vi "Data to XY Plot GPIB.vi"(7 "String of Data":string) -> (8 "XY Graph":cluster{sgl[], sgl[]}(graph))   [LabVIEW 2024, in "Keithley 648X Series.lvlib"]
doc: "Sends a default command string to the instrument whenever a new VISA session is opened, or the instrument is reset. Use this VI as a subVI for the <b>Initialize</b> and <b>Reset</b> VIs. Altering this VI could cause these two VIs to operate incorrectly."
uses:
  <instrlib>/Keithley 648X Series/Keithley 648X Series.lvlib
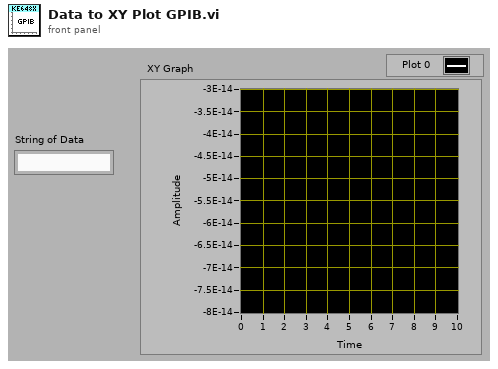
[diagram p1: front panel]
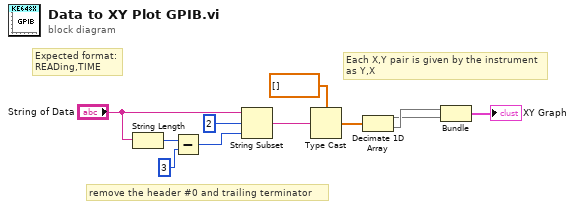
[diagram p0: block diagram]
diagram:
  # "remove the header #0 and trailing terminator"
  # "Each X,Y pair is given by the instrument\nas Y,X"
  # "Expected format:\nREADing,TIME"
  n1 = String Length(string="String of Data") -> (length=w11:i32)
  n2 = Subtract(x=w11, y=3) -> (x-y=w7:i32)
  n3 = String Subset(string="String of Data", offset (0)=2 ("x"), length (rest)=w7) -> (substring=w6:string)
  n4 = Type Cast(type=sgl[] [], x=w6) -> (*(type *) &x=w4:sgl[])
  n5 = Decimate 1D Array(w4) -> (w1:sgl[], w2:sgl[])
  n6 = Bundle(w2, w1) -> (→"XY Graph":cluster{sgl[], sgl[]})  [unwired: 1 in]
